vi "AssertsLess.vi"(0 "VI Reference In":refnum<vi>, 1 "Label (VI Title)":string="Default", 11 "error in (no error)":errorcluster) -> (4 "VI Reference Out":refnum<vi>, 15 "error out":errorcluster)   [LabVIEW 2016, in "Drona Test.lvlib"]
uses:
  Drona Test.lvlib
  main/apis/Stimulus/KeyBoardSimulation/ValueSignalLatchBooleanString.vi
  main/apis/Assert/AssertControlValue/Less.vi
  <vilib>/addons/_JKI Toolkits/Caraya/classes/Assert/Assert Error.vi
  <vilib>/addons/_JKI Toolkits/Caraya/classes/Assert/Assert Not Error.vi
  main/apis/Assert/AssertControlValue/LessOrEqual.vi
  <vilib>/addons/_JKI Toolkits/Caraya/classes/Test/Test.lvclass
  main/Drona.lvlib
  <vilib>/addons/_JKI Toolkits/Caraya/classes/Assert/Assert.lvclass
  main/apis/Stimulus/KeyBoardSimulation/KeyboardSimulation.lvlib
  main/apis/Assert/AssertControlValue/AssertControlValue.lvlib
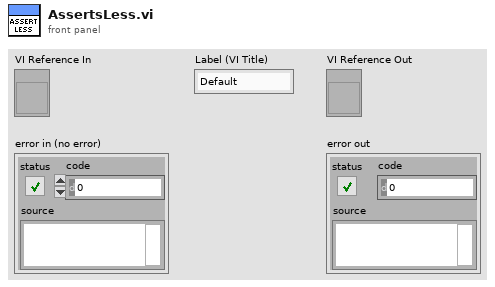
[diagram p1: front panel]
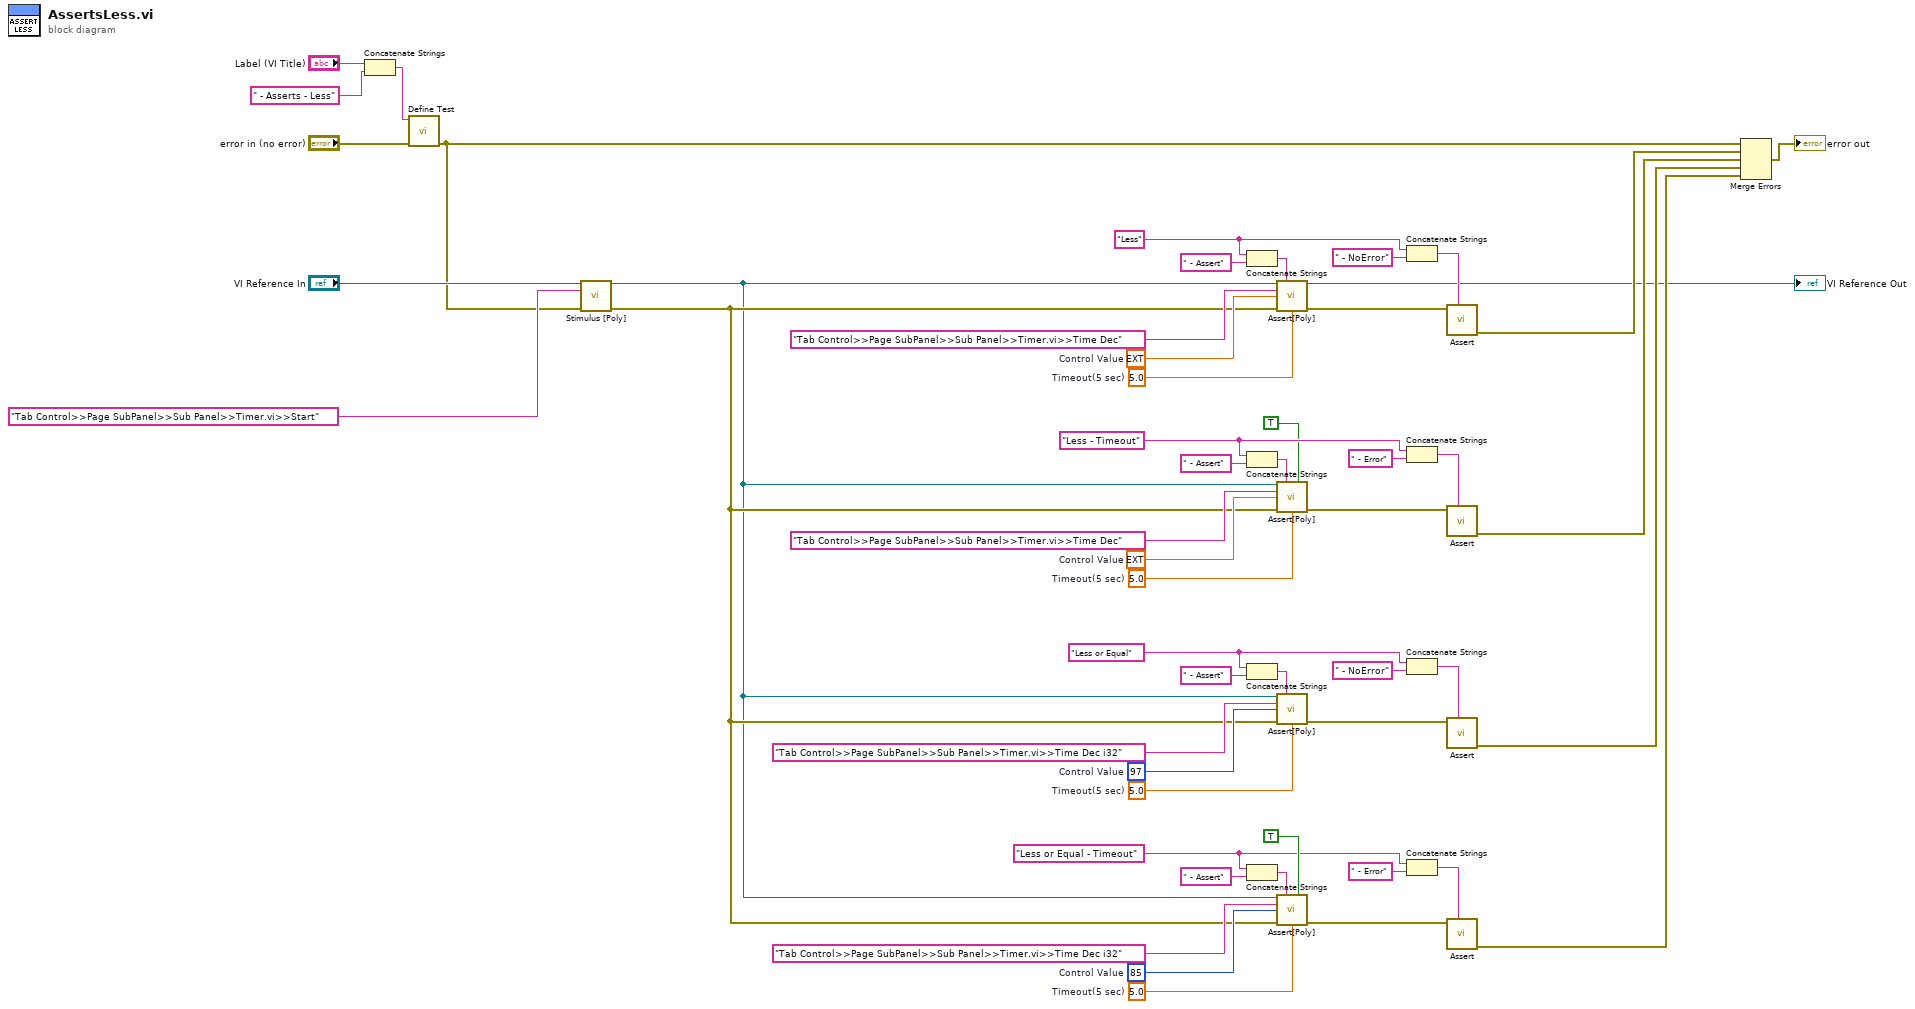
[diagram p0: block diagram]
diagram:
  w35 = 5.0  # Timeout(5 sec)
  w34 = 97  # Control Value
  w33 = "Less or Equal" ("string")
  w36 = 5.0  # Timeout(5 sec)
  w37 = 85  # Control Value
  w38 = "Less or Equal - Timeout" ("string")
  w18 = 5.0  # Timeout(5 sec)
  w19 = ext 97.0  # Control Value
  w20 = "Less" ("string")
  w17 = 5.0  # Timeout(5 sec)
  w16 = ext 85.0  # Control Value
  w15 = "Less - Timeout" ("string")
  n1 = Concatenate Strings("Label (VI Title)", " - Asserts - Less" ("Label (VI Title)")) -> (w49:string)
  n2 = call <vilib>:"Define Test.vi"("error in (no error)"="error in (no error)", "Label (VI Title)"=w49) -> ("error out"=w46:errorcluster)  [unwired: 9 in]
  n3 = call-poly "Stimulus [Poly].vi"("VI Reference In"="VI Reference In", "Control Path"="Tab Control>>Page SubPanel>>Sub Panel>>Timer.vi>>Start", "error in"=w46) -> ("VI Reference Out"=w6:refnum<vi>, "error out"=w7:errorcluster)  [unwired: 11 in]
  n4 = Concatenate Strings(w20, " - Assert" ("string")) -> (w22:string)
  n5 = Concatenate Strings(w15, " - Assert" ("string")) -> (w13:string)
  n6 = Concatenate Strings(w33, " - Assert" ("string")) -> (w31:string)
  n7 = Concatenate Strings(w38, " - Assert" ("string")) -> (w40:string)
  n8 = call-poly "Assert[Poly].vi"("VI Reference In"=w6, "Label"=w22, "Control Path"="Tab Control>>Page SubPanel>>Sub Panel>>Timer.vi>>Time Dec", "Control Value"=w19, "Error In"=w7, "Timeout(5 sec)"=w18) -> ("VI Reference Out"=→"VI Reference Out":refnum<vi>, "Error Out"=w23:errorcluster)  [unwired: 8 in]
  n9 = call-poly "Assert[Poly].vi"("VI Reference In"=w6, "Label"=w13, "Assert Only? (F)"=TRUE, "Control Path"="Tab Control>>Page SubPanel>>Sub Panel>>Timer.vi>>Time Dec", "Control Value"=w16, "Error In"=w7, "Timeout(5 sec)"=w17) -> ("Error Out"=w12:errorcluster)  [unwired: 7 in, 1 out]
  n10 = call-poly "Assert[Poly].vi"("VI Reference In"=w6, "Label"=w31, "Control Path"="Tab Control>>Page SubPanel>>Sub Panel>>Timer.vi>>Time Dec i32", "Control Value"=w34, "Error In"=w7, "Timeout(5 sec)"=w35) -> ("Error Out"=w30:errorcluster)  [unwired: 8 in, 1 out]
  n11 = call-poly "Assert[Poly].vi"("VI Reference In"=w6, "Label"=w40, "Assert Only? (F)"=TRUE, "Control Path"="Tab Control>>Page SubPanel>>Sub Panel>>Timer.vi>>Time Dec i32", "Control Value"=w37, "Error In"=w7, "Timeout(5 sec)"=w36) -> ("Error Out"=w41:errorcluster)  [unwired: 7 in, 1 out]
  n12 = Concatenate Strings(w20, " - NoError" ("string")) -> (w21:string)
  n13 = Concatenate Strings(w15, " - Error" ("string")) -> (w14:string)
  n14 = Concatenate Strings(w33, " - NoError" ("string")) -> (w32:string)
  n15 = Concatenate Strings(w38, " - Error" ("string")) -> (w39:string)
  n16 = call-poly <vilib>:"Assert.vi"("Label"=w21, "Not Error?"=w23) -> ("error out"=w5:errorcluster)  [unwired: 9 in]
  n17 = call-poly <vilib>:"Assert.vi"("Label"=w14, "Error?"=w12) -> ("error out"=w4:errorcluster)  [unwired: 9 in]
  n18 = call-poly <vilib>:"Assert.vi"("Label"=w32, "Not Error?"=w30) -> ("error out"=w3:errorcluster)  [unwired: 9 in]
  n19 = call-poly <vilib>:"Assert.vi"("Label"=w39, "Error?"=w41) -> ("error out"=w2:errorcluster)  [unwired: 9 in]
  n20 = Merge Errors(w46, w5, w4, w3, w2) -> (→"error out":errorcluster)
